vi "_FPGA_DDS_CycleAccumulator.vi"(0 "Conj.InitCyc*2^32":u64, 1 "Conj1":cluster{"Ratio*2^15":u16, "CycleDiff":u64}[](array[cluster])=[{"Ratio*2^15"=0, "CycleDiff"=0}, {"Ratio*2^15"=0, "CycleDiff"=0}, {"Ratio*2^15"=0, "CycleDiff"=0}, {"Ratio*2^15"=0, "CycleDiff"=0}, {"Ratio*2^15"=0, "CycleDiff"=0}, {"Ratio*2^15"=0, "CycleDiff"=0}, {"Ratio*2^15"=0, "CycleDiff"=0}, {"Ratio*2^15"=0, "CycleDiff"=0}, {"Ratio*2^15"=0, "CycleDiff"=0}, {"Ratio*2^15"=0, "CycleDiff"=0}], 2 "Conj2":cluster{"Ratio*2^15":u16, "CycleDiff":u64}[](array[cluster])=[{"Ratio*2^15"=0, "CycleDiff"=0}, {"Ratio*2^15"=0, "CycleDiff"=0}, {"Ratio*2^15"=0, "CycleDiff"=0}, {"Ratio*2^15"=0, "CycleDiff"=0}, {"Ratio*2^15"=0, "CycleDiff"=0}, {"Ratio*2^15"=0, "CycleDiff"=0}, {"Ratio*2^15"=0, "CycleDiff"=0}, {"Ratio*2^15"=0, "CycleDiff"=0}, {"Ratio*2^15"=0, "CycleDiff"=0}, {"Ratio*2^15"=0, "CycleDiff"=0}], 4 "DeCycle*U32":u32, 5 "1/DeCyc*2^8":u32, 6 "Conj1.#":u8, 7 "Init_strobe":bool, 8 "Conj2.#":u8, 9 "ConjSelector":bool, 11 "SlowCycle":bool) -> (12 "Conj?":bool, 14 "TheFirstConj?":bool, 15 "Cycle_U64":u64, 16 "Conj.Cyc":u64, 17 "CycleDiff?":u64, 18 "Actual DeCycle":u32, 19 "ConjIndex":u8)   [LabVIEW 2018]
uses:
  <instrlib>/_niInstr/Basic Elements/v1/FPGA/niInstr Basic Elements v1 FPGA.lvlib
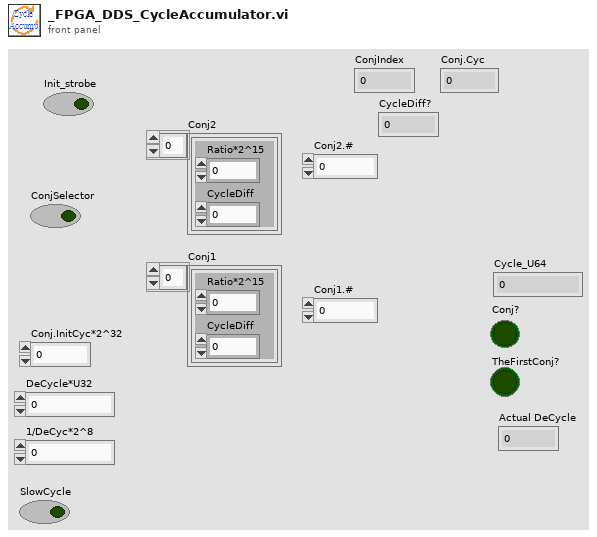
[diagram p1: front panel]
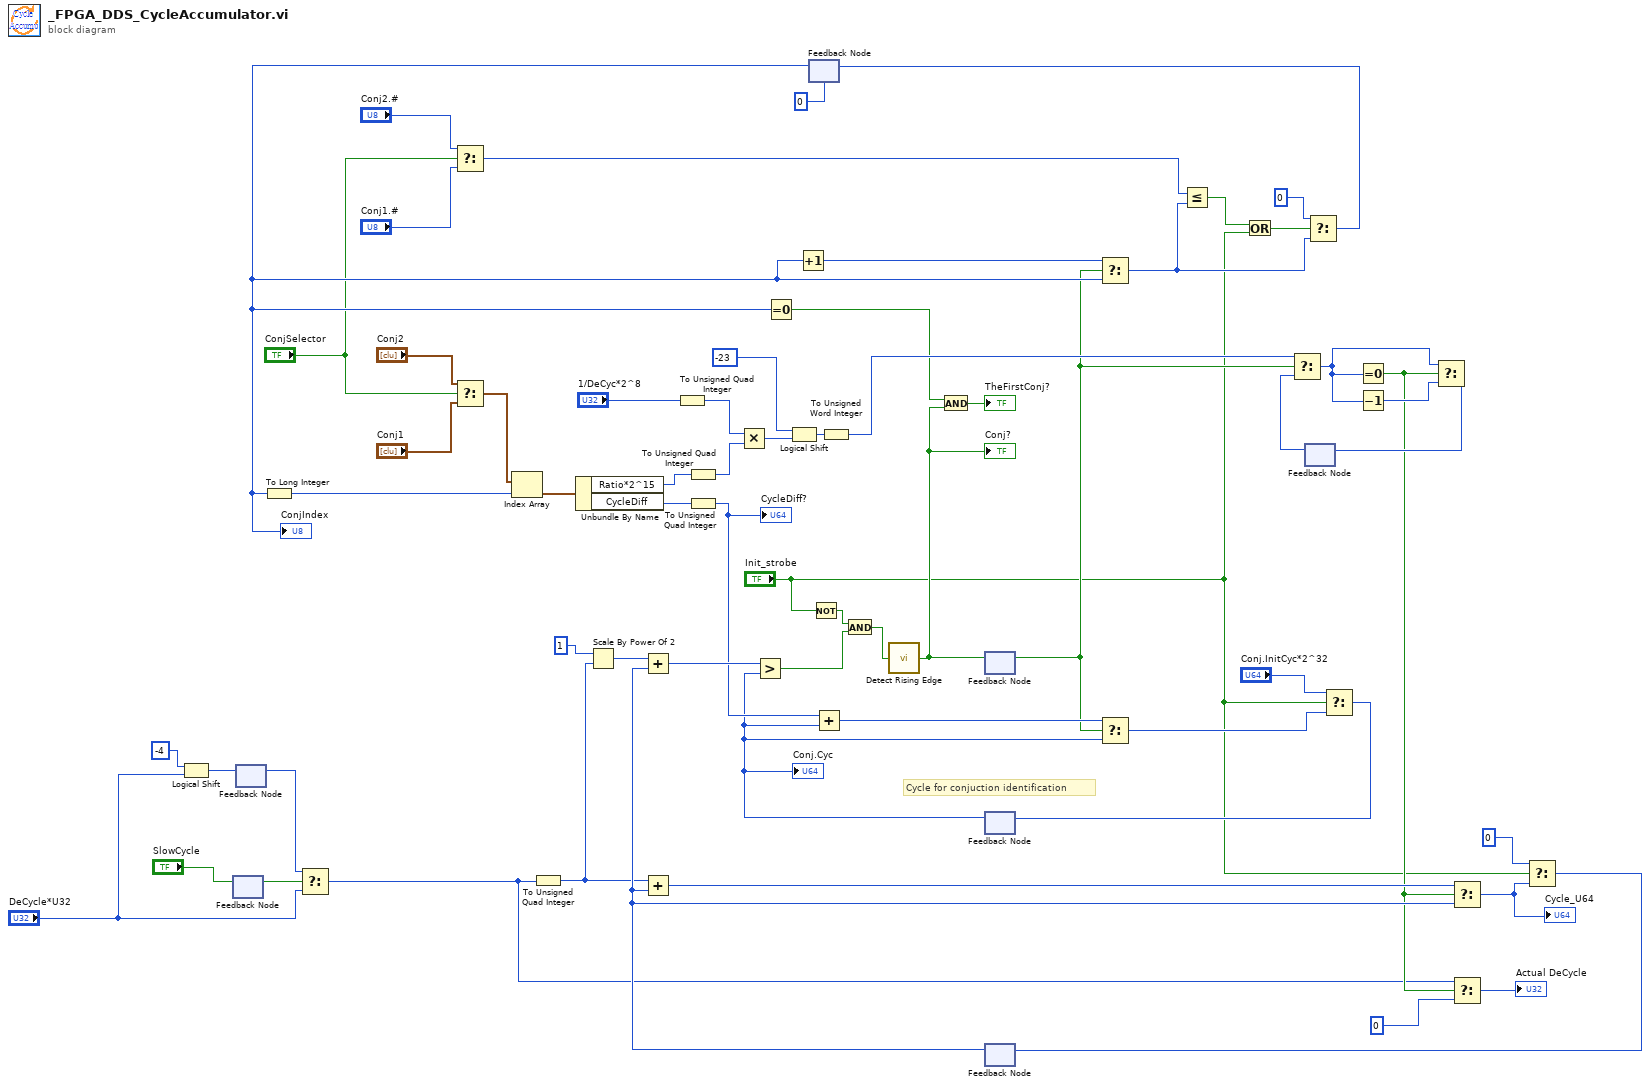
[diagram p0: block diagram]
diagram:
  # "Cycle for conjuction identification"
  n1 = Logical Shift(y=i16 -4 ("n"), x="DeCycle*U32") -> (x << y=w51:u32)
  n2 = feedback #1() -> (w18:bool)  [unwired: 1 in]
  n3 = feedback-in #1("SlowCycle") -> ()
  n4 = feedback-in #2(w51) -> ()
  n5 = feedback #2() -> (w23:u32)  [unwired: 1 in]
  n6 = Select(t=w23, s=w18, f="DeCycle*U32") -> (s? t:f=w8:u32)
  n7 = Select(t="Conj2.#", s="ConjSelector", f="Conj1.#") -> (s? t:f=w25:u8)
  n8 = Select(t="Conj2", s="ConjSelector", f="Conj1") -> (s? t:f=w28:cluster{"Ratio*2^15":u16, "CycleDiff":u64}[])
  n9 = To Unsigned Quad Integer(1:w8) -> (0:w11:u64)
  n10 = Scale By Power Of 2(n=i16 1 ("y"), x=w11) -> (x*2^n=w21:u64)
  n11 = To Unsigned Quad Integer(1:"1/DeCyc*2^8") -> (0:w55:u64)
  n12 = feedback #3(u8 0) -> (w32:u8)
  "ConjIndex" <- w32
  n13 = To Long Integer(number=w32) -> (32bit integer=w61:i32)
  n14 = Index Array(array=w28, index=w61) -> (element=w60:cluster{"Ratio*2^15":u16, "CycleDiff":u64})
  n15 = Unbundle By Name(w60) -> ("Ratio*2^15"=w58:u16, "CycleDiff"=w59:u64)
  n16 = To Unsigned Quad Integer(1:w58) -> (0:w57:u64)
  n17 = To Unsigned Quad Integer(1:w59) -> (0:w7:u64)
  "CycleDiff?" <- w7
  n18 = Multiply(x=w55, y=w57) -> (x*y=w54:u64)
  n19 = Equal To 0?(x=w32) -> (x = 0?=w31:bool)
  n20 = Logical Shift(y=i16 -23, x=w54) -> (x << y=w49:u64)
  n21 = Increment(x=w32) -> (x+1=w45:u8)
  n22 = Not(x="Init_strobe") -> (.not. x?=w5:bool)
  n23 = To Unsigned Word Integer(number=w49) -> (unsigned 16bit integer=w36:u16)
  n24 = feedback #4() -> (w16:bool)  [unwired: 1 in]
  n25 = feedback #5() -> (w6:u64)  [unwired: 1 in]
  "Conj.Cyc" <- w6
  n26 = Add(x=w7, y=w6) -> (x+y=w63:u64)
  n27 = feedback #6() -> (w14:u64)  [unwired: 1 in]
  n28 = Add(x=w21, y=w14) -> (x+y=w20:u64)
  n29 = Add(x=w11, y=w14) -> (x+y=w15:u64)
  n30 = Greater?(x=w20, y=w6) -> (0:w3:bool)
  n31 = And(x=w5, y=w3) -> (x .and. y?=w2:bool)
  n32 = call <instrlib>:"Detect Rising Edge.vi"("signal"=w2) -> ("edge detected"=w17:bool)  [unwired: 14 in]
  "Conj?" <- w17
  n33 = And(x=w31, y=w17) -> (x .and. y?=→"TheFirstConj?":bool)
  n34 = feedback-in #4(w17) -> ()
  n35 = Select(t=w45, s=w16, f=w32) -> (s? t:f=w44:u8)
  n36 = Select(t=w63, s=w16, f=w6) -> (s? t:f=w37:u64)
  n37 = Less Or Equal?(x=w25, y=w44) -> (x <= y?=w33:bool)
  n38 = Or(x=w33, y="Init_strobe") -> (x .or. y?=w34:bool)
  n39 = feedback #7() -> (w46:u16)  [unwired: 1 in]
  n40 = Select(t=w36, s=w16, f=w46) -> (s? t:f=w40:u16)
  n41 = Select(t=u8 0, s=w34, f=w44) -> (s? t:f=w42:u8)
  n42 = feedback-in #3(w42) -> ()
  n43 = Select(t="Conj.InitCyc*2^32", s="Init_strobe", f=w37) -> (s? t:f=w38:u64)
  n44 = feedback-in #5(w38) -> ()
  n45 = Equal To 0?(x=w40) -> (x = 0?=w12:bool)
  n46 = Decrement(x=w40) -> (x-1=w41:u16)
  n47 = Select(t=w40, s=w12, f=w41) -> (s? t:f=w47:u16)
  n48 = feedback-in #7(w47) -> ()
  n49 = Select(t=w15, s=w12, f=w14) -> (s? t:f=w13:u64)
  "Cycle_U64" <- w13
  n50 = Select(t=w8, s=w12, f=u32 0) -> (s? t:f=→"Actual DeCycle":u32)
  n51 = Select(t=u64 0, s="Init_strobe", f=w13) -> (s? t:f=w1:u64)
  n52 = feedback-in #6(w1) -> ()
